vi "Get Base Command.vi"(8 "error in (no error)":errorcluster, 11 "RST in":refnum<class "RST.lvclass">) -> (0 "error out":errorcluster, 2 "Base Command":string, 3 "RST out":refnum<class "RST.lvclass">)   [LabVIEW 2023, in "HAF.lvlib" / "RST.lvclass"]
doc: "Returns the base command whch is used to build up the overall command string – parameters will be added to this as necessary.  The framework will add the line terminator \\n.\n\nSubclasses MUST override this member and must not add a line terminator on the end of the command; on this class an error is returned."
uses:
  RST.lvclass
  RST.lvclass/RST.ctl
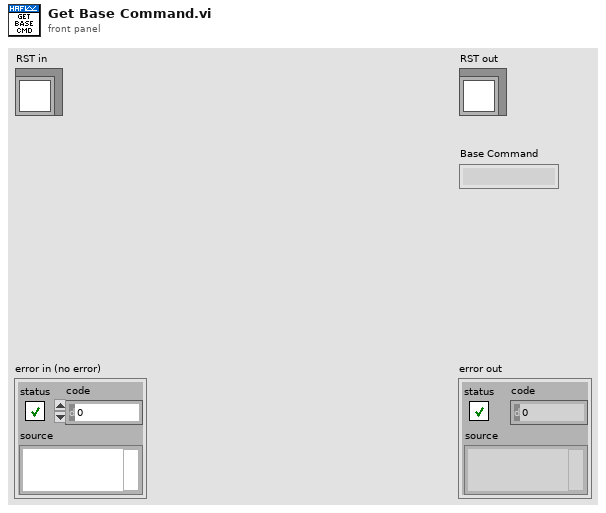
[diagram p1: front panel]
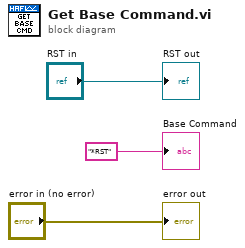
[diagram p0: block diagram]
diagram:
  "error out" <- "error in (no error)"
  "RST out" <- "RST in"
  "Base Command" <- "*RST" ("Base Command")
